vi "Read Frequency.vi"(8 "error in (no error)":errorcluster, 11 "Attack in":refnum<class "Net Attack.lvclass">) -> (0 "error out":errorcluster, 2 "Frequency":i32, 3 "Attack out":refnum<class "Net Attack.lvclass">)   [LabVIEW 2014, in "Net Attack.lvclass"]
uses:
  Net Attack.lvclass
  Net Attack.lvclass/Net Attack.ctl
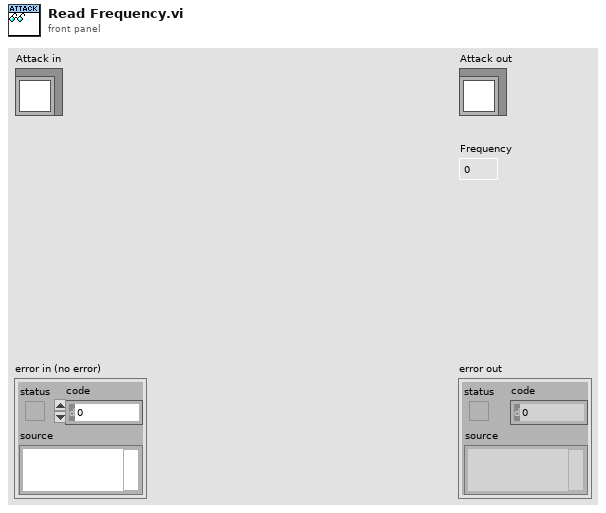
[diagram p1: front panel]
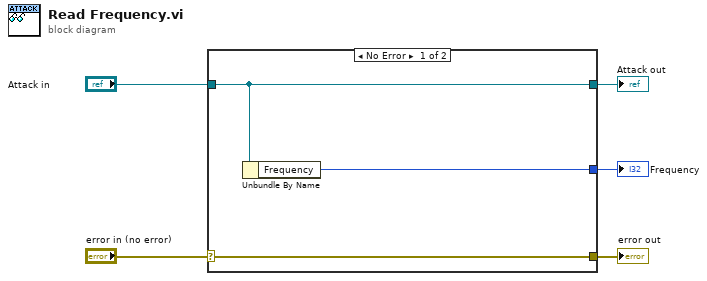
[diagram p0: block diagram]
diagram:
  n1 = case shown="No Error" "error in (no error)" {
    selector: "error in (no error)" -> [w8 w9]
    tunnel: [w8 w9] -> w4
    tunnel: [w7 w10] -> w2
    tunnel: "Attack in" -> [w7 w10]
    tunnel: [w6 _] -> w1
    frame No Error {
      n2 = Unbundle By Name(w7) -> ("Frequency"=w6:i32)
    }
    frame Error {
    }
  }
  "error out" <- w4
  "Attack out" <- w2
  "Frequency" <- w1
